vi "constrain_axes.vi"(8 "error in":errorcluster, 9 "Axis current positions":dbl[](array[numeric])=[0.0, 0.0, 0.0, 0.0, 0.0, 0.0], 11 "Axis positions in":dbl[](array[numeric])=[0.0, 0.0, 0.0, 0.0, 0.0, 0.0]) -> (0 "error out":errorcluster, 1 "In range":bool, 3 "Axis positions out":dbl[](array[numeric]))   [LabVIEW 2024]
uses:
  <vilib>/Analysis/coordinate.llb/Angle Units.ctl
  <vilib>/Analysis/coordinate.llb/Wrap Angle (scalar).vi
  <vilib>/Analysis/NI_AAL_Angle.lvlib
panel:
  in  "Axis ranges":dbl[](array[numeric])=[75.0, 75.0, 45.0, 200.0, 200.0, 10.0]
  # "Optional.  Specifying current position\nprevents flip-flopping near 180 degrees."
  # "Wrap the angles of the rotation axes into the canonical range and check the axis ranges, coercing to the limits."
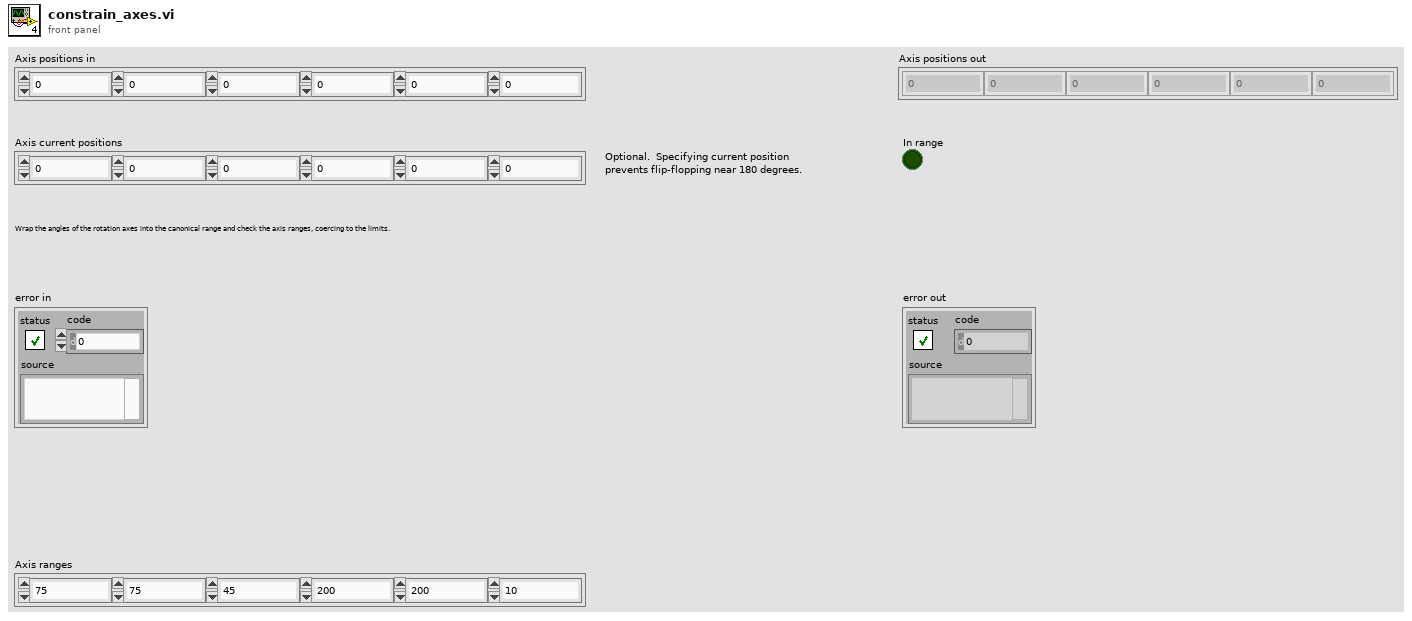
[diagram p1: front panel]
types:
  T1 = typedef "NI_AAL_Angle.lvlib/Angle Units.ctl" = i32
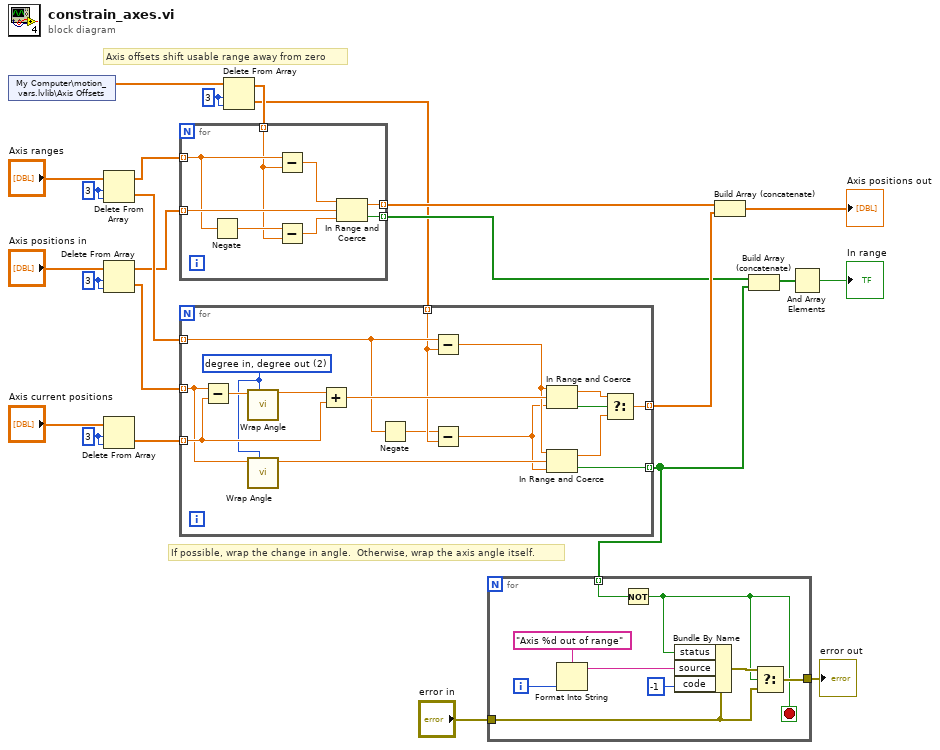
[diagram p0: block diagram]
diagram:
  w4 = 3 ("length")
  w19 = 3 ("length")
  w21 = 3 ("length")
  w23 = 3 ("length")
  # "Axis offsets shift usable range away from zero"
  # "If possible, wrap the change in angle.  Otherwise, wrap the axis angle itself."
  n1 = shared-variable "My Computer\\motion_vars.lvlib\\Axis Offsets"() -> (w1:dbl[])  [unwired: 1 in, 1 out]
  n2 = Delete From Array(array="Axis ranges", length=w19, index=w19) -> (deleted portion=w17:dbl[], array with subset deleted=w16:dbl[])
  n3 = Delete From Array(array="Axis positions in", length=w23, index=w23) -> (deleted portion=w24:dbl[], array with subset deleted=w15:dbl[])
  n4 = Delete From Array(array="Axis current positions", length=w21, index=w21) -> (deleted portion=w14:dbl[])  [unwired: 1 out]
  n5 = Delete From Array(array=w1, length=w4, index=w4) -> (deleted portion=w2:dbl[], array with subset deleted=w3:dbl[])
  n6 = for {
    tunnel: w16 -> [w29] mode=indexing
    tunnel: w15 -> [w32] mode=indexing
    tunnel: [w31] -> w8 mode=indexing
    tunnel: [w30] -> w13 mode=indexing
    tunnel: w3 -> [w26] mode=indexing
    n7 = Negate(x=w29) -> (-x=w27:dbl)
    n8 = Subtract(x=w29, y=w26) -> (x-y=w28:dbl)
    n9 = Subtract(x=w27, y=w26) -> (x-y=w25:dbl)
    n10 = In Range and Coerce(upper limit=w28, x=w32, lower limit=w25) -> (coerced(x)=w30:dbl, In Range?=w31:bool)
  }
  n11 = for {
    tunnel: w24 -> [w40] mode=indexing
    tunnel: w17 -> [w37] mode=indexing
    tunnel: w14 -> [w47] mode=indexing
    tunnel: [w42] -> w12 mode=indexing
    tunnel: [w41] -> w5 mode=indexing
    tunnel: w2 -> [w35] mode=indexing
    w39 = T1 2 items=["radian in, radian out", "radian in, degree out", "degree in, degree out", "degree in, radian out"] ("angle units")
    n12 = Subtract(x=w40, y=w47) -> (x-y=w49:dbl)
    n13 = call-poly <vilib>:"Wrap Angle.vi"("angle units"=w39, "angle in"=w49) -> ("angle out"=w48:dbl)  [unwired: 8 in, 1 out]
    n14 = call-poly <vilib>:"Wrap Angle.vi"("angle units"=w39, "angle in"=w40) -> ("angle out"=w38:dbl)  [unwired: 8 in, 1 out]
    n15 = Add(x=w48, y=w47) -> (x+y=w46:dbl)
    n16 = Negate(x=w37) -> (-x=w34:dbl)
    n17 = Subtract(x=w37, y=w35) -> (x-y=w36:dbl)
    n18 = Subtract(x=w34, y=w35) -> (x-y=w33:dbl)
    n19 = In Range and Coerce(upper limit=w36, x=w46, lower limit=w33) -> (coerced(x)=w44:dbl, In Range?=w45:bool)
    n20 = In Range and Coerce(upper limit=w36, x=w38, lower limit=w33) -> (coerced(x)=w43:dbl, In Range?=w41:bool)
    n21 = Select(t=w44, s=w45, f=w43) -> (s? t:f=w42:dbl)
  }
  n22 = for {
    tunnel: [w56] -> w10
    tunnel: "error in" -> [w55]
    tunnel: w5 -> [w54] mode=indexing
    i -> [w50]
    stop <- w53 stop-if-true
    n23 = Format Into String(format string="Axis %d out of range" ("source"), w50) -> (resulting string=w52:string)  [unwired: 2 in, 1 out]
    n24 = Not(x=w54) -> (.not. x?=w53:bool)
    n25 = Bundle By Name(cluster=w55, "status"=w53, "source"=w52, "code"=-1) -> (w58:errorcluster)
    n26 = Select(t=w58, s=w53, f=w55) -> (s? t:f=w56:errorcluster)
  }
  "error out" <- w10
  n27 = Build Array (concatenate)(w13, w12) -> (→"Axis positions out":dbl[])
  n28 = Build Array (concatenate)(w8, w5) -> (w7:bool[])
  n29 = And Array Elements(Boolean array=w7) -> (logical AND=→"In range":bool)
